vi "QuestionAsked.vi"(8 "Error In":errorcluster, 10 "Question":string, 11 "reference in":refnum<class "Wolfram.lvclass">) -> (0 "Error Out":errorcluster, 3 "reference out":refnum<class "Wolfram.lvclass">)   [LabVIEW 2020, in "Wolfram.lvclass"]
uses:
  Wolfram.lvclass
  <vilib>/httpClient/LabVIEWHTTPClient.lvlib
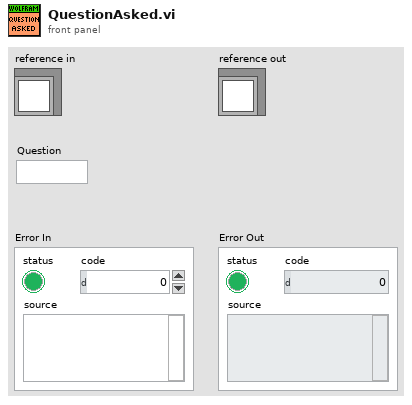
[diagram p1: front panel]
types:
  T1 = typedef "Wolfram.lvclass/ObjectAttributes.ctl" = cluster{"AnswerRef":refnum<vi>}
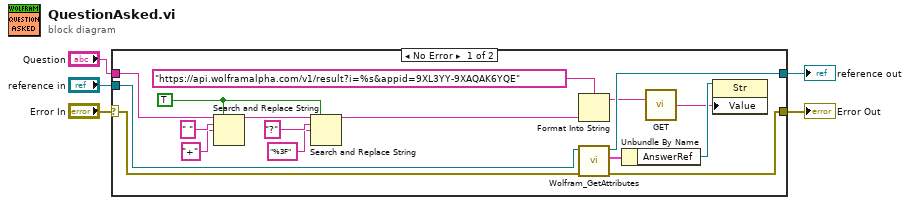
[diagram p0: block diagram]
diagram:
  n1 = case shown="No Error" "Error In" {
    selector: "Error In" -> [w22 w24]
    tunnel: [w20 w24] -> w4
    tunnel: [w18 w23] -> w2
    tunnel: "reference in" -> [w19 w23]
    tunnel: "Question" -> [w9 _]
    frame No Error {
      w10 = TRUE ("ignore case? (F)")
      n2 = Search and Replace String(replace all?=w10, input string=w9, search string=" ", replace string="+" ("replace string (\"\")")) -> (result string=w14:string)  [unwired: 4 in, 3 out]
      n3 = Search and Replace String(replace all?=w10, input string=w14, search string="?", replace string="%3F" ("replace string (\"\")")) -> (result string=w11:string)  [unwired: 4 in, 3 out]
      n4 = Format Into String(format string="https://api.wolframalpha.com/v1/result?i=%s&appid=9XL3YY-9XAQAK6YQE" ("url"), w11) -> (resulting string=w8:string)  [unwired: 2 in, 1 out]
      n5 = call "Wolfram_GetAttributes.vi"("error in (no error)"=w22, "reference in"=w19) -> ("error out"=w20:errorcluster, "Data"=w21:T1, "reference out"=w18:refnum<class "Wolfram.lvclass">)  [unwired: 6 in, 1 out]
      n6 = Unbundle By Name(w21) -> ("AnswerRef"=w7:refnum<vi>)
      n7 = call <vilib>:"GET.vi"("url"=w8) -> ("body"=w6:string)  [unwired: 11 in, 3 out]
      n8 = property class="Str"(reference=w7, "Value"=w6) -> ()  [unwired: 1 in, 2 out]
    }
    frame Error {
    }
  }
  "Error Out" <- w4
  "reference out" <- w2
